vi "set_laser_onoff.vi"(8 "error in (no error)":errorcluster, 10 "on?":bool=TRUE, 11 "LightSourceMH110125Tsunami in":refnum<class "LightSourceMH110125Tsunami.lvclass">) -> (0 "error out":errorcluster, 3 "LightSourceMH110125Tsunami out":refnum<class "LightSourceMH110125Tsunami.lvclass">)   [LabVIEW 2010, in "LightSourceMH110125Tsunami.lvclass"]
uses:
  LightSourceMH110125Tsunami.lvclass
panel:
  out "percentage warm":dbl
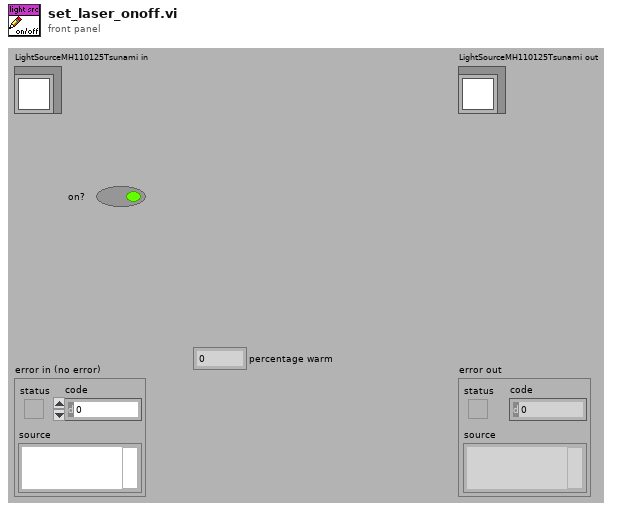
[diagram p1: front panel]
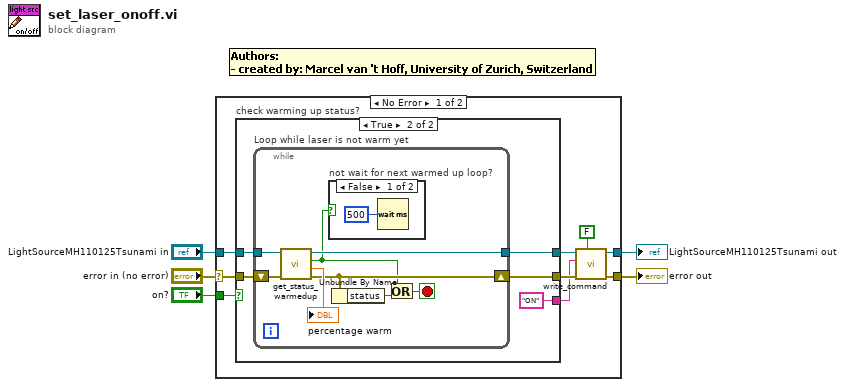
[diagram p0: block diagram]
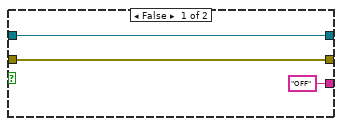
[diagram p2: hidden frame]
diagram:
  n1 = case shown="No Error" "error in (no error)" {
    selector: "error in (no error)" -> [w8 w33]
    tunnel: [w13 w33] -> w1
    tunnel: [w14 w32] -> w2
    tunnel: "LightSourceMH110125Tsunami in" -> [w10 w32]
    tunnel: "on?" -> [w11 _]
    frame No Error {
      n2 = case "check warming up status?" shown="True" w11 {
        tunnel: w10 -> [w17 w22]
        tunnel: w8 -> [w16 w21]
        tunnel: [w17 w20] -> w9
        tunnel: [w16 w19] -> w7
        tunnel: ["OFF" ("string to write") "ON" ("string to write")] -> w6
        frame False {
        }
        frame True {
          n3 = while "Loop while laser is not warm yet" {
            tunnel: w22 -> [w29]
            tunnel: [w28] -> w20
            shift-right: [w26] -> w19
            shift-left: w21 -> [w30]
            stop <- w24 stop-if-true
            n4 = call-dynamic "get_status_warmedup.vi"("error in (no error)"=w30, "LightSourceMH110125Tsunami in"=w29) -> ("error out"=w26:errorcluster, "percentage warm"=→"percentage warm":dbl, "warmed up?"=w23:bool, "LightSourceMH110125Tsunami out"=w28:refnum<class "LightSourceMH110125Tsunami.lvclass">)  [unwired: 6 in]
            n5 = case "not wait for next warmed up loop?" shown="False" w23 {
              frame False {
                n6 = Wait (ms)(milliseconds to wait=u32 500) -> ()  [unwired: 1 out]
              }
              frame True {
              }
            }
            n7 = Unbundle By Name(w26) -> ("status"=w25:bool)
            n8 = Or(x=w23, y=w25) -> (x .or. y?=w24:bool)
          }
        }
      }
      n9 = call-dynamic "write_command.vi"("error in (no error)"=w7, "read (T)"=FALSE, "string to write"=w6, "LightSourceMH110125Tsunami in"=w9) -> ("error out"=w13:errorcluster, "LightSourceMH110125Tsunami out"=w14:refnum<class "LightSourceMH110125Tsunami.lvclass">)  [unwired: 5 in, 1 out]
    }
    frame Error {
    }
  }
  "error out" <- w1
  "LightSourceMH110125Tsunami out" <- w2
